vi "Memory.Pointer.Read.Subset.In Place.Safe (1D U8).vi"(7 "length":i64 format="%d bytes", 8 "error in (no error)":errorcluster, 9 "offset (0)":i64 format="%d bytes", 10 "buffer in":u8[](array[numeric]) format="%02x", 11 "Pointer in":refnum<class "Memory.Pointer.lvclass">) -> (0 "error out":errorcluster, 1 "offset dup":i64 format="%d bytes", 2 "buffer out":u8[](array[numeric]) format="%02x", 3 "Pointer out":refnum<class "Memory.Pointer.lvclass">)   [LabVIEW 2016, in "LabVIEW Memory Manager.lvlib" / "Memory.Pointer.lvclass"]
uses:
  Memory.Pointer.lvclass
  Memory.Pointer.Offset to Address.Unsafe.vi
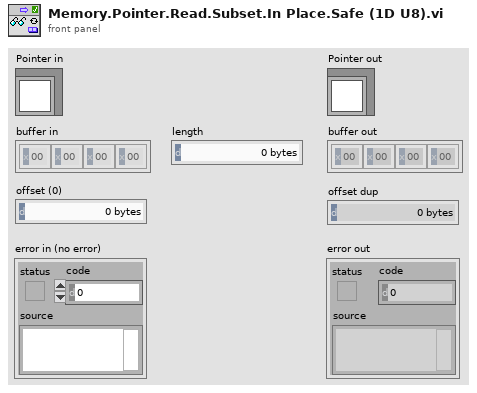
[diagram p1: front panel]
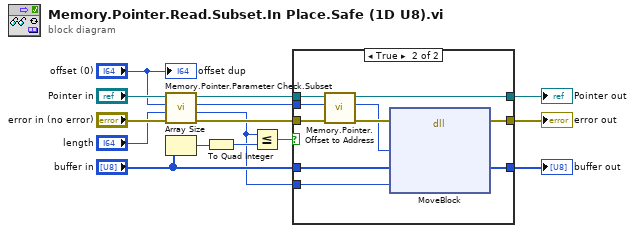
[diagram p0: block diagram]
diagram:
  n1 = call "Memory.Pointer.Parameter Check.Subset.vi"("error in (no error)"="error in (no error)", "length"="length", "offset"="offset (0)", "Pointer in"="Pointer in") -> ("error out"=w6:errorcluster, "length out"=w2:i64, "offset out"=w4:i64, "Pointer out"=w7:refnum<class "Memory.Pointer.lvclass">)  [unwired: 3 in, 1 out]
  n2 = Array Size(array="buffer in") -> (size(s)=w13:i32)
  n3 = To Quad Integer(1:w13) -> (0:w5:i64)
  n4 = Less Or Equal?(x=w2, y=w5) -> (x <= y?=w1:bool)
  n5 = case shown="True" w1 {
    tunnel: [w18 w27] -> w15
    tunnel: [w17 w26] -> w14
    tunnel: [w16 w25] -> w9
    tunnel: w7 -> [w18 w24]
    tunnel: w6 -> [w17 w23]
    tunnel: w4 -> [_ w22]
    tunnel: "buffer in" -> [w16 w21]
    tunnel: w2 -> [_ w20]
    frame False {
      # "#TODO\nThrow error."
    }
    frame True {
      n6 = call-poly "Memory.Pointer.Offset to Address.vi"("error in (no error)"=w23, "offset"=w22, "Pointer in"=w24) -> ("error out"=w28:errorcluster, "address"=w19:u64, "Pointer out"=w27:refnum<class "Memory.Pointer.lvclass">)  [unwired: 6 in]
      n7 = dll-call lib="LabVIEW" fn="MoveBlock"(error in=w28, "src pointer"=w19, "dst pointer"=w21, "size"=w20) -> (error out=w26:errorcluster, "dst pointer"=w25:u8[])  [unwired: 5 in, 1 out]
    }
  }
  "error out" <- w14
  "Pointer out" <- w15
  "buffer out" <- w9
  "offset dup" <- "offset (0)"
